vi "test_Bitfile Reload_Scalars.vi"(8 "error in (no error)":errorcluster, 11 "TestCase in":refnum<class "FPGA Addon Bitfile Reload Unit Tests.lvclass">=refnum) -> (0 "error out":errorcluster, 3 "TestCase out":refnum<class "FPGA Addon Bitfile Reload Unit Tests.lvclass">)   [LabVIEW 2026, in "FPGA Addon Bitfile Reload Unit Tests.lvclass"]
uses:
  FPGA Addon Bitfile Reload Unit Tests.lvclass
  APIs/Scripting API/TypeDefs/Output Scalar Data.ctl
  APIs/Scripting API/Scripting API.lvlib
  FPGA Addon Test Class/FPGA Addon Test Class.lvclass
  Addon/Addon System Explorer/FPGA Addon System Explorer.lvlib
  APIs/Scripting API/Public/Bitfile Resources/Import Bitfile Scalars (Instances)/Import Scalars - all.vi
  Addon/Addon Shared/Types/FPGA Addon Data Type.ctl
  Addon/Addon Shared/FPGA Addon Shared.lvlib
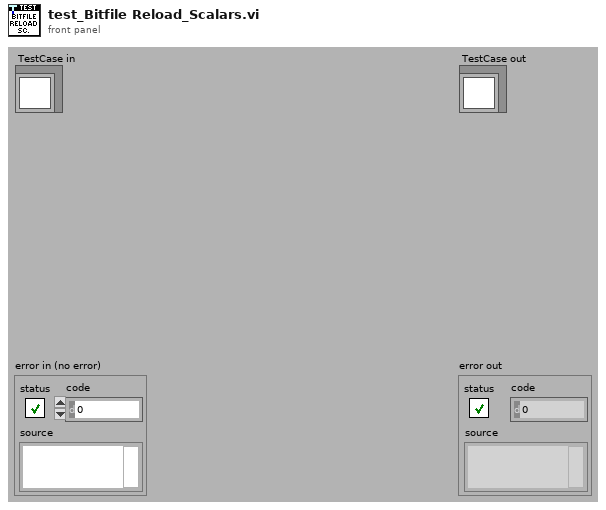
[diagram p1: front panel]
types:
  T1 = typedef "Scripting API.lvlib/Output Scalar Data.ctl" = cluster{"Bitfile Name":string, "SysDef Channel Name":string, "Imported":bool, "Data Type":T2}
  T2 = typedef "FPGA Addon Shared.lvlib/FPGA Addon Data Type.ctl" = enum8{"<Null>", "I8", "I16", "I32", "I64", "U8", "U16", "U32", "U64", "SGL", "Boolean", "Analog PWM In Settings", "Analog PWM In", "Digital PWM In Settings", "Digital PWM In", "Digital PWM Out", "Sine Out", "FXP", "FXP+/-24.5", "FXP+/-16.5", "FXP+/-32.8", "FXP+/-64.32", "FXP+/-16.7", "FXP+/-20.5", "FXP+/-27.5", "FXP+/-32.16", "FXP+16.3", "FXP+18.3", "Digital Static In", "Digital Static Out", "Digital Static In Settings", "Digital WSS Out", "Quad Encoder Settings", "Quad Encoder In", "Group"}
  T3 = typedef "Custom Device API.lvlib/Custom Device Item Ref.ctl" = u64
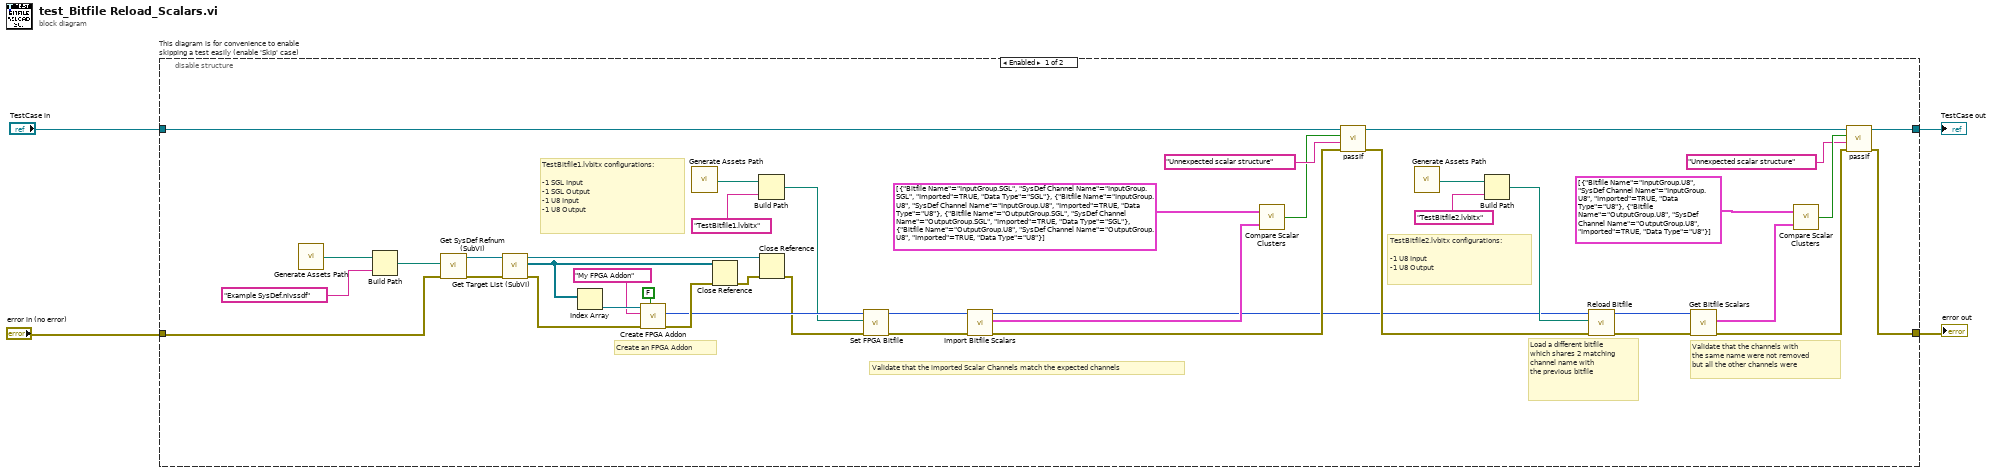
[diagram p0: block diagram]
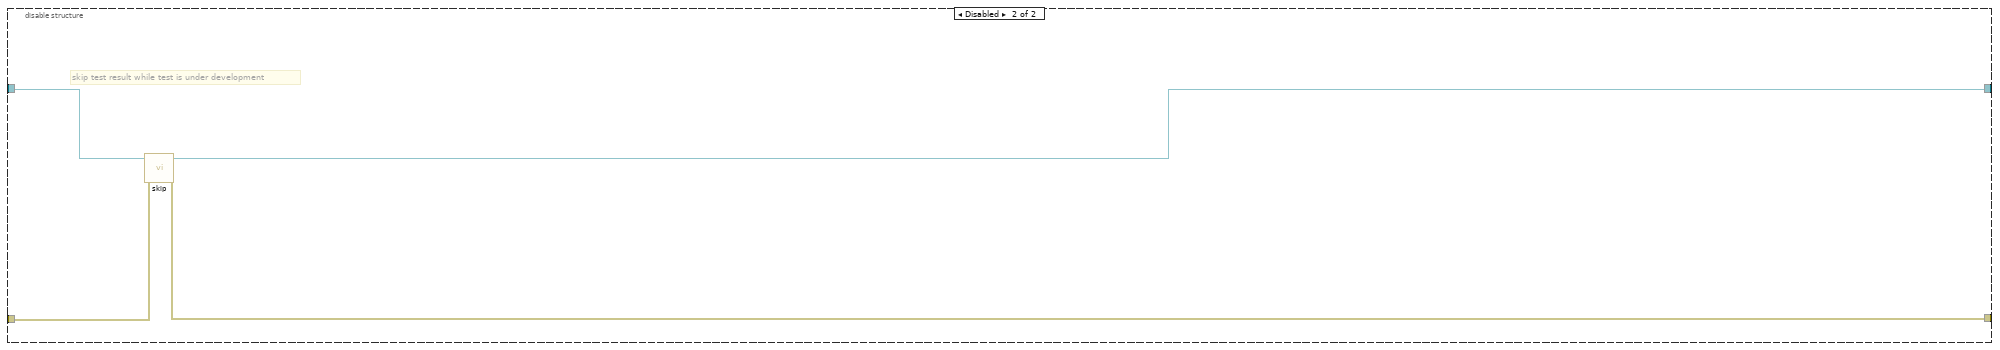
[diagram p2: hidden frame]
diagram:
  n1 = disable-structure "This diagram is for convenience to enable skipping a test easily (enable 'Skip' case)" shown="Enabled" {
    disable-tunnel: "TestCase in" -> [w10 w50]
    disable-tunnel: [w8 w48] -> w1
    disable-tunnel: [w7 w49] -> w3
    disable-tunnel: "error in (no error)" -> [w9 w47]
    frame Enabled {
      # "TestBitfile2.lvbitx configurations:\n\n-1 U8 Input\n-1 U8 Output"
      # "TestBitfile1.lvbitx configurations:\n\n-1 SGL Input\n-1 SGL Output\n-1 U8 Input\n-1 U8 Output"
      # "Validate that the channels with \nthe same name were not removed\nbut all the other channels were"
      # "Load a different bitfile\nwhich shares 2 matching\nchannel name with \nthe previous bitfile"
      # "Validate that the imported Scalar Channels match the expected channels"
      # "Create an FPGA Addon"
      n2 = call "Generate Assets Path.vi"() -> ("Assets path"=w26:path)
      n3 = Build Path(base path=w26, name or relative path="Example SysDef.nivssdf") -> (appended path=w45:path)
      n4 = call "Get SysDef Refnum (SubVI).vi"("error in (no error)"=w9, "System Definition path"=w45) -> ("error out"=w41:errorcluster, "NationalInstruments.VeriStand.SystemDefinitionAPI.SystemDefinition"=w44:refnum<k39>)  [unwired: 8 in]
      n5 = call "Get Target List (SubVI).vi"("error in (no error)"=w41, "NationalInstruments.VeriStand.SystemDefinitionAPI.SystemDefinition"=w44) -> ("error out"=w40:errorcluster, "Target List Refnums"=w39:refnum<k39>[], "NationalInstruments.VeriStand.SystemDefinitionAPI.SystemDefinition"=w38:refnum<k39>)  [unwired: 7 in]
      n6 = Index Array(array=w39) -> (element=w43:refnum<k39>)  [unwired: 1 in]
      n7 = call "Create FPGA Addon.vi"("group scalars"=FALSE, "error in"=w40, "FPGA addon name"="My FPGA Addon", "NationalInstruments.VeriStand.SystemDefinitionAPI.Target"=w43) -> ("error out"=w36:errorcluster, "FPGA addon refnum"=w34:T3)  [unwired: 5 in, 1 out]
      n8 = call "Generate Assets Path.vi"() -> ("Assets path"=w25:path)
      n9 = Close Reference(reference=w39, error in (no error)=w36) -> (error out=w37:errorcluster)
      n10 = Build Path(base path=w25, name or relative path="TestBitfile1.lvbitx") -> (appended path=w31:path)
      n11 = Close Reference(reference=w38, error in (no error)=w37) -> (error out=w33:errorcluster)
      n12 = call "Set FPGA Bitfile.vi"("error in"=w33, "FPGA bitfile path"=w31, "FPGA addon refnum in"=w34) -> ("error out"=w30:errorcluster, "FPGA addon refnum out"=w29:T3)  [unwired: 7 in]
      n13 = call-poly "Import Bitfile Scalars.vi"("error in"=w30, "FPGA addon refnum in"=w29) -> ("error out"=w28:errorcluster, "imported bitfile scalars out"=w23:T1[], "FPGA addon refnum out"=w18:T3)  [unwired: 7 in]
      n14 = call "Compare Scalar Clusters.vi"("Target bitfile scalars in"=w23, "Reference bitfile scalars in"=T1[] [{"Bitfile Name"="InputGroup.SGL", "SysDef Channel Name"="InputGroup.SGL", "Imported"=TRUE, "Data Type"=enum."SGL"}, {"Bitfile Name"="InputGroup.U8", "SysDef Channel Name"="InputGroup.U8", "Imported"=TRUE, "Data Type"=enum."U8"}, {"Bitfile Name"="OutputGroup.SGL", "SysDef Channel Name"="OutputGroup.SGL", "Imported"=TRUE, "Data Type"=enum."SGL"}, {"Bitfile Name"="OutputGroup.U8", "SysDef Channel Name"="OutputGroup.U8", "Imported"=TRUE, "Data Type"=enum."U8"}] ("bitfile scalars out")) -> ("Equal ?"=w24:bool)
      n15 = call-dynamic "passIf.vi"("error in (no error)"=w28, "message (\"\")"="Unnexpected scalar structure" ("message (\"\")"), "pass"=w24, "TestCase in"=w10) -> ("error out"=w20:errorcluster, "TestCase out"=w15:refnum<class "FPGA Addon Bitfile Reload Unit Tests.lvclass">)  [unwired: 6 in]
      n16 = call "Generate Assets Path.vi"() -> ("Assets path"=w21:path)
      n17 = Build Path(base path=w21, name or relative path="TestBitfile2.lvbitx") -> (appended path=w19:path)
      n18 = call "Reload Bitfile.vi"("error in (no error)"=w20, "NewVal"=w19, "Item Ref in"=w18) -> ("error out"=w17:errorcluster, "Section Ref out"=w16:T3)  [unwired: 7 in]
      n19 = call "Get Bitfile Scalars.vi"("error in"=w17, "FPGA addon refnum in"=w16) -> ("error out"=w13:errorcluster, "bitfile scalars out"=w14:T1[])  [unwired: 7 in, 1 out]
      n20 = call "Compare Scalar Clusters.vi"("Target bitfile scalars in"=w14, "Reference bitfile scalars in"=T1[] [{"Bitfile Name"="InputGroup.U8", "SysDef Channel Name"="InputGroup.U8", "Imported"=TRUE, "Data Type"=enum."U8"}, {"Bitfile Name"="OutputGroup.U8", "SysDef Channel Name"="OutputGroup.U8", "Imported"=TRUE, "Data Type"=enum."U8"}] ("imported bitfile scalars out")) -> ("Equal ?"=w12:bool)
      n21 = call-dynamic "passIf.vi"("error in (no error)"=w13, "message (\"\")"="Unnexpected scalar structure" ("message (\"\")"), "pass"=w12, "TestCase in"=w15) -> ("error out"=w7:errorcluster, "TestCase out"=w8:refnum<class "FPGA Addon Bitfile Reload Unit Tests.lvclass">)  [unwired: 6 in]
    }
    frame Disabled {
      # "skip test result while test is under development"
      n22 = call <vilib>:"skip.vi"("error in (no error)"=w47, "TestCase in"=w50) -> ("error out"=w49:errorcluster, "TestCase out"=w48:refnum<class "FPGA Addon Bitfile Reload Unit Tests.lvclass">)  [unwired: 8 in]
    }
  }
  "error out" <- w3
  "TestCase out" <- w1
